vi "Query Error Count.vi"(0 "VISA resource name":refnum<visa-resource-name>, 11 "error in (no error)":errorcluster) -> (4 "VISA resource name out":refnum<visa-resource-name>, 6 "Error Count":i32, 15 "error out":errorcluster)   [LabVIEW 2018, in "XP Power PLS600.lvlib"]
doc: "Returns the number of Errors/Events in the Errors/Events Queue."
uses:
  XP Power PLS600.lvlib
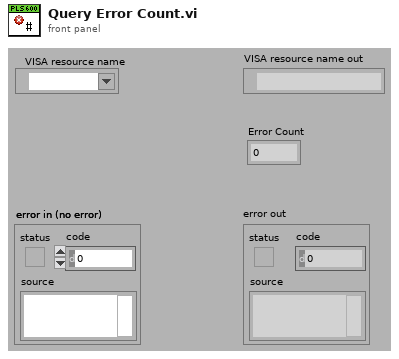
[diagram p1: front panel]
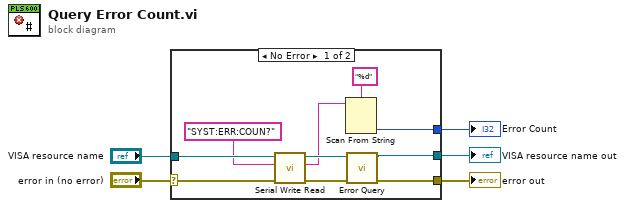
[diagram p0: block diagram]
diagram:
  n1 = case shown="No Error" "error in (no error)" {
    selector: "error in (no error)" -> [w12 w16]
    tunnel: "VISA resource name" -> [w13 w17]
    tunnel: [w14 w17] -> w4
    tunnel: [w15 w16] -> w3
    tunnel: [w6 _] -> w1
    frame No Error {
      n2 = call "Serial Write Read.vi"("error in (no error)"=w12, "Write Buffer"="SYST:ERR:COUN?" ("Command to Send (empty)"), "VISA resource name"=w13) -> ("error out"=w11:errorcluster, "Read Buffer"=w7:string, "VISA resource name out"=w10:refnum<visa-resource-name>)  [unwired: 6 in]
      n3 = Scan From String(format string="%d", input string=w7) -> (output 1=w6:i32)  [unwired: 3 in, 3 out]
      n4 = call "Error Query.vi"("error in (no error)"=w11, "VISA resource name"=w10) -> ("error out"=w15:errorcluster, "VISA resource name out"=w14:refnum<visa-resource-name>)  [unwired: 6 in, 2 out]
    }
    frame Error {
    }
  }
  "error out" <- w3
  "VISA resource name out" <- w4
  "Error Count" <- w1
